vi "Stop Core.vi"(10 "final error code":i32, 11 "Grid Screen in":refnum<class "Grid Screen.lvclass">) -> (3 "Grid Screen out":refnum<class "Grid Screen.lvclass">)   [LabVIEW 2021, in "Grid Screen.lvlib" / "Grid Screen.lvclass"]
doc: "<p>(<strong>Filename</strong>: <span class=\"dnl\">Actor Framework.lvlib:Actor.lvclass:Stop Core.vi</span>)</p>\n<p>Defines what the actor does before it stops. Use the <strong>final error code</strong> input to determine whether the actor shut down in response to an error.</p>\n<p>By default, this method passes the Stop message along to all <a href=\"nihelplauncher://docs/csh?context=lvcore_lvcomm_af_launch_nested_actor\">auto-stop nested actors</a>. A descendant class may override this method to define additional behavior, such as shutting down any processes the actor initiated in its override of the <a href=\"nihelplauncher://docs/csh?context=lvcore_lvcomm_af_actor_core\">Actor Core</a> method.</p>"
uses:
  Grid Screen.lvclass
  Grid Screen.lvclass/Grid Screen.ctl
  <vilib>/ActorFramework/Actor/Actor.lvclass
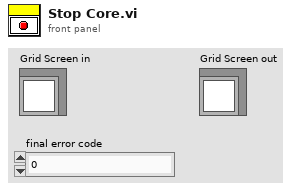
[diagram p1: front panel]
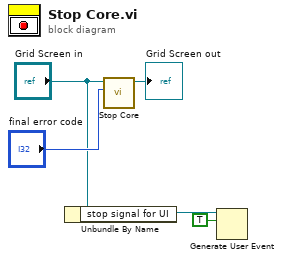
[diagram p0: block diagram]
diagram:
  n1 = Unbundle By Name("Grid Screen in") -> ("stop signal for UI"=w2:refnum<user-event>)
  n2 = call-parent "Stop Core.vi"("final error code"="final error code", "Actor in"="Grid Screen in") -> ("Actor out"=→"Grid Screen out":refnum<class "Grid Screen.lvclass">)  [unwired: 9 in]
  n3 = Generate User Event(user event=w2, event data cluster=TRUE ("event data")) -> ()  [unwired: 2 in, 2 out]
